vi "Advanced VI Analysis.vi"() -> ()   [LabVIEW 2023]
doc: "This example uses the advanced VI Analyzer VIs to perform an analysis on an LLB of VIs. The \"New Task\" VI uses preset test settings loaded from a CFG file that was created from the VI Analyzer user interface. Certain advanced VIs are used to perform tasks like adding an LLB to the analysis, removing a single VI from the analysis, removing certain tests from the analysis, and modifying a configuration value on one test. Once the analysis performed by \"VIAn Run.vi\" is complete, the \"VIAn Easy Report.vi\" saves the analysis results to an HTML report."
uses:
  <vilib>/Platform/browser.llb/Open URL in Default Browser (path).vi
  <vilib>/addons/analyzer/NI_VIAnalyzerTKVIs.lvlib
panel:
  in  "Tests with ten maximum failures":string[](array[string])=["Coercion Dots", "Spell Check"]
  out "VI in Analysis":string
  out "Analysis Progress":dbl(slide) scale=0.0..100.0
  out "Tests Run":string[](array[string])
  out "VIs Tested":path[](array[path])
  in  "Modified Value":T1={"Test Name"="VI Documentation", "Control Name"="Control Description", "Control Value"=FALSE}
  in  "VI to Remove":string="Container VI.vi"
  in  "Excluded Tests":string[](array[string])=["Enabled Debugging", "Panel Size and Position"]
  # "Overview: Demonstrates the use of the VI Analyzer and VI Analyzer Utility VIs to customize a programmatic analysis.\nRequirements: VI Analyzer Toolkit\nInstructions:\nRun the VI."
  # "Exclude these tests from the VI Analyzer Task."
  # "Set these tests to have 10 maximum failures for the VI Analyzer Task."
  # "Remove the top-level placeholder VI from the analysis."
  # "Disable the option on the \"VI Documentation\" test to analyze control descriptions."
  # "Show the progress of the analysis."
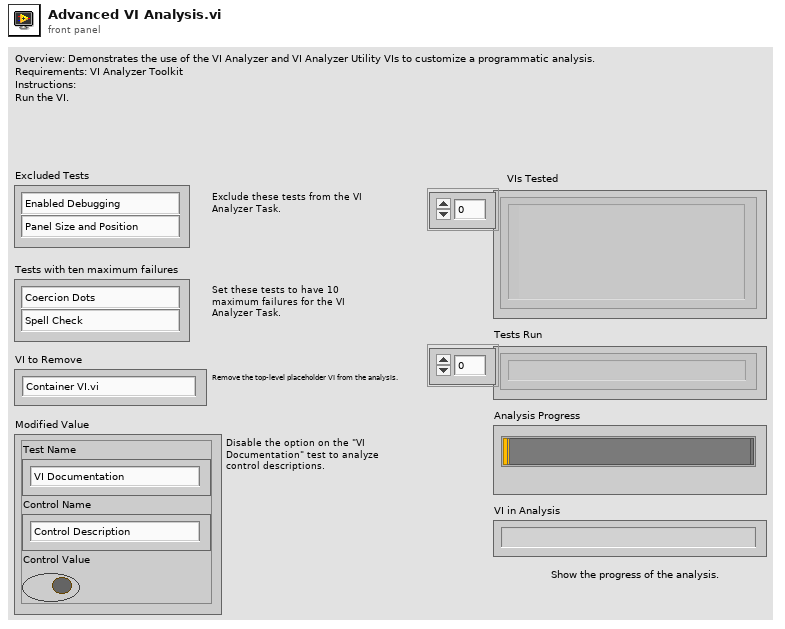
[diagram p1: front panel]
types:
  T1 = cluster{"Test Name":string, "Control Name":string, "Control Value":bool}
  T2 = typedef "VIAnAPI Ref.ctl" = refnum<k1>
  T3 = typedef "VIAnCtl API Test Config Data.ctl" = cluster{"Test Ranking":T4, "Max Failures":u32, "Control Values":T5[], "Run Test?":bool}
  T4 = typedef "VIAnCtl TestRanking.ctl" = u16
  T5 = typedef "VIAnCtl Config Control Value.ctl" = cluster{"Control Name":string, "Control Value":variant}
  T6 = typedef "VIAnCtl Results.ctl" = cluster{"Test Name":string, "Results Data":T7[], "Status":T8, "Exceed Max Fails?":bool}
  T7 = typedef "VIAnCtl ResultsData (index).ctl" = cluster{"Result Message":string, "Ref Index":i32}
  T8 = typedef "VIAnCtl ResultStatus.ctl" = enum16{"Pass", "Fail", "Skipped", "VI not loadable", "Test not loadable", "Test not runnable", "Test error out"}
  T9 = typedef "VIAnRes Parsed Results Data (by VI).ctl" = cluster{"VI Path":path, "Pass":cluster{"row":i32, "column":i32}[], "Fail":cluster{"row":i32, "column":i32}[], "Skipped":cluster{"row":i32, "column":i32}[], "VI not loadable":cluster{"row":i32, "column":i32}[], "Test not loadable":cluster{"row":i32, "column":i32}[], "Test not runnable":cluster{"row":i32, "column":i32}[], "Test error out":cluster{"row":i32, "column":i32}[]}
  T10 = typedef "VIAnRes Parsed Results Data (by Test).ctl" = cluster{"Test Name":string, "Pass":cluster{"VI Path":path, "index":cluster{"row":i32, "column":i32}}[], "Fail":cluster{"VI Path":path, "index":cluster{"row":i32, "column":i32}}[], "Skipped":cluster{"VI Path":path, "index":cluster{"row":i32, "column":i32}}[]}
  T11 = typedef "VIAnCtl Test Config Data.ctl" = cluster{"Test Name":string, "Config Ref":refnum<vi>, "Ref Valid?":bool, "Test Ranking":T4, "Max Failures":u32, "Test Path":path, "Control Values":T5[], "Selected?":bool}
  T12 = cluster{"Raw Results":T6[][], "Parsed Results Data (by VI)":T9[], "Parsed Results Data (by Test)":T10[], "Summary Statistics":cluster{"Passed Tests":i32, "Failed Tests":i32, "Skipped Tests":i32, "VIs not loadable":i32, "Tests not loadable":i32, "Tests not runnable":i32, "Test error out":i32, "Start Time":u32, "Total Time (s)":dbl}, "Test Config Data":T11[]}
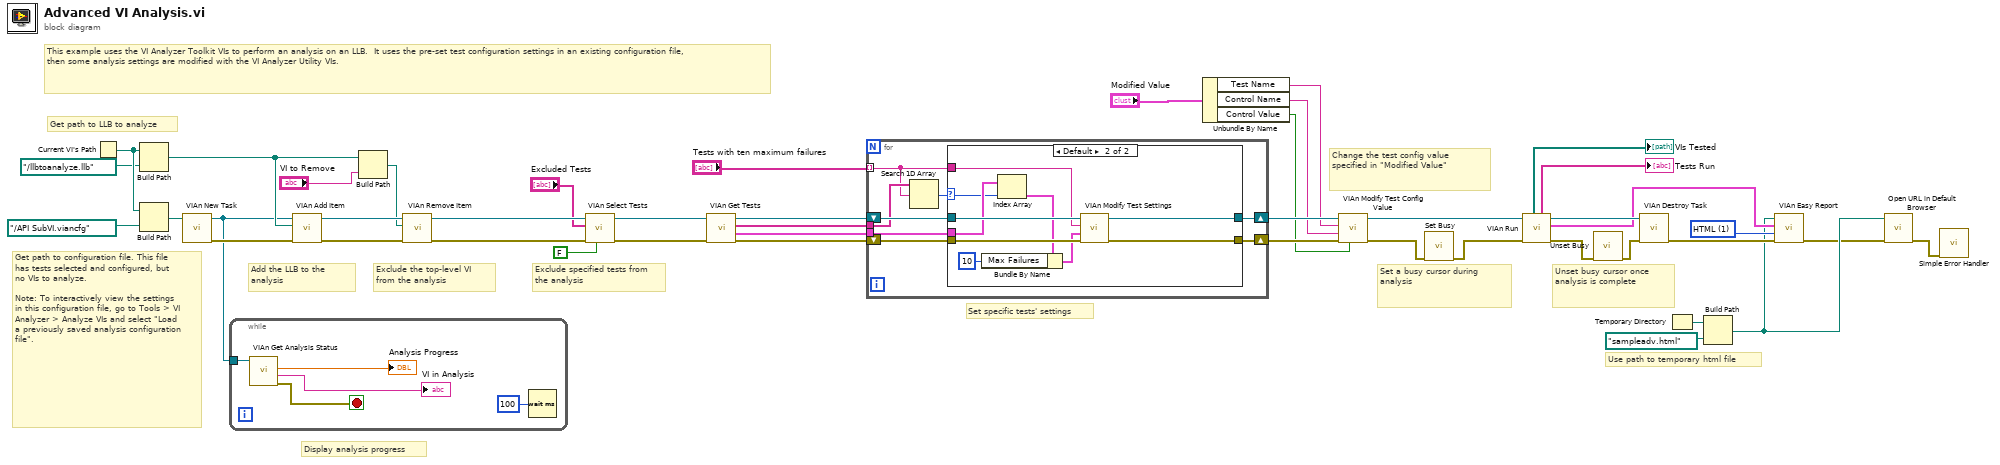
[diagram p0: block diagram]
diagram:
  w32 = u16 1 items=["ASCII", "HTML", "RSL File"] ("Report Save Type (ASCII)")
  # "Set specific tests' settings"
  # "Exclude specified tests from the analysis"
  # "Display analysis progress"
  # "Unset busy cursor once analysis is complete"
  # "Set a busy cursor during analysis"
  # "Get path to LLB to analyze"
  # "This example uses the VI Analyzer Toolkit VIs to perform an analysis on an LLB.  It uses the pre-set test configuration settings in an existing configuration file, then some analysis settings are modified with the VI Analyzer Utility VIs."
  # "Use path to temporary html file"
  # "Change the test config value specified in \"Modified Value\""
  # "Get path to configuration file. This file has tests selected and configured, but no VIs to analyze.\n\nNote: To interactively view the settings in this configuration file, go to Tools > VI Analyzer > Analyze VIs and select \"Load a previously saved analysis configuration file\"."
  # "Exclude the top-level VI from the analysis"
  # "Add the LLB to the analysis"
  n1 = Current VI's Path() -> (path=w41:path)
  n2 = Build Path(base path=w41, name or relative path=path "../llbtoanalyze.llb" ("path")) -> (appended path=w37:path)
  n3 = Build Path(base path=w41, name or relative path=path "../API SubVI.viancfg" ("path")) -> (appended path=w44:path)
  n4 = call <vilib>:"VIAn New Task.vi"("Path to Configuration File"=w44) -> ("error out"=w42:errorcluster, "VI Analyzer Task"=w15:T2)  [unwired: 2 in, 7 out]
  n5 = while {
    tunnel: w15 -> [w49]
    stop <- w45 stop-if-true
    n6 = call <vilib>:"VIAn Get Analysis Status.vi"("VI Analyzer Task in"=w49) -> ("error out"=w45:errorcluster, "VI in Analysis"=→"VI in Analysis":string, "Percent Complete"=→"Analysis Progress":dbl)  [unwired: 1 in, 7 out]
    n7 = Wait (ms)(milliseconds to wait=u32 100) -> ()  [unwired: 1 out]
  }
  n8 = call <vilib>:"VIAn Add Item.vi"("error in (no error)"=w42, "Item to Add"=w37, "VI Analyzer Task in"=w15) -> ("error out"=w38:errorcluster, "VI Analyzer Task out"=w39:T2)  [unwired: 7 out]
  n9 = Build Path(base path=w37, name or relative path="VI to Remove") -> (appended path=w36:path)
  n10 = call <vilib>:"VIAn Remove Item.vi"("error in (no error)"=w38, "Item to Remove"=w36, "VI Analyzer Task in"=w39) -> ("error out"=w12:errorcluster, "VI Analyzer Task out"=w14:T2)  [unwired: 7 out]
  n11 = call <vilib>:"VIAn Select Tests.vi"("Select Test? (T)"=FALSE, "error in (no error)"=w12, "Test Names"="Excluded Tests", "VI Analyzer Task in"=w14) -> ("error out"=w9:errorcluster, "VI Analyzer Task out"=w10:T2)  [unwired: 6 out]
  n12 = call <vilib>:"VIAn Get Tests.vi"("error in (no error)"=w9, "VI Analyzer Task in"=w10) -> ("error out"=w8:errorcluster, "Test Configurations"=w6:T3[], "Test Names"=w5:string[], "VI Analyzer Task out"=w7:T2)  [unwired: 6 out]
  n13 = for {
    shift-right: [w54] -> w30
    shift-left: w8 -> [w56]
    shift-right: [w55] -> w31
    shift-left: w7 -> [w57]
    tunnel: "Tests with ten maximum failures" -> [w52] mode=indexing
    tunnel: w6 -> [w50]
    tunnel: w5 -> [w53]
    n14 = Search 1D Array(1D array=w53, element=w52) -> (index of element=w51:i32)  [unwired: 1 out]
    n15 = case shown="Default" w51 {
      selector: w51 -> [_ w62]
      tunnel: w57 -> [w59 w69]
      tunnel: w56 -> [w58 w68]
      tunnel: [w59 w67] -> w55
      tunnel: [w58 w66] -> w54
      tunnel: w52 -> [_ w64]
      tunnel: w50 -> [_ w63]
      frame -1 {
      }
      frame Default {
        n16 = Index Array(array=w63, index=w62) -> (element=w61:T3)
        n17 = Bundle By Name(cluster=w61, "Max Failures"=u32 10) -> (w65:T3)
        n18 = call <vilib>:"VIAn Modify Test Settings.vi"("error in (no error)"=w68, "New Test Info"=w65, "Test Name"=w64, "VI Analyzer Task in"=w69) -> ("error out"=w66:errorcluster, "VI Analyzer Task out"=w67:T2)  [unwired: 6 out]
      }
    }
  }
  n19 = Unbundle By Name("Modified Value") -> ("Test Name"=w27:string, "Control Name"=w26:string, "Control Value"=w25:bool)
  n20 = call <vilib>:"VIAn Modify Test Config Value.vi"("Control Value"=w25, "error in (no error)"=w30, "Control Name"=w26, "Test Name"=w27, "VI Analyzer Task in"=w31) -> ("error out"=w19:errorcluster, "VI Analyzer Task out"=w20:T2)  [unwired: 5 out]
  n21 = call <vilib>:"Set Busy.vi"("error in (no error)"=w19) -> ("error out"=w18:errorcluster)  [unwired: 3 in, 7 out]
  n22 = call <vilib>:"VIAn Run.vi"("error in (no error)"=w18, "VI Analyzer Task in"=w20) -> ("error out"=w17:errorcluster, "Analysis Results"=w33:T12, "VI Analyzer Task out"=w35:T2, "Tests Run"=→"Tests Run":string[], "VIs Tested"=→"VIs Tested":path[])  [unwired: 5 out]
  n23 = call <vilib>:"Unset Busy.vi"("error in (no error)"=w17) -> ("error out"=w16:errorcluster)  [unwired: 1 in, 9 out]
  n24 = call <vilib>:"VIAn Destroy Task.vi"("error in (no error)"=w16, "VI Analyzer Task in"=w35) -> ("error out"=w34:errorcluster)  [unwired: 9 out]
  n25 = Temporary Directory() -> (w24:path)
  n26 = Build Path(base path=w24, name or relative path=path "sampleadv.html" ("path")) -> (appended path=w3:path)
  n27 = call <vilib>:"VIAn Easy Report.vi"("error in (no error)"=w34, "Report Save Type (ASCII)"=w32, "Analysis Results"=w33, "Report Save Path"=w3) -> ("error out"=w2:errorcluster)  [unwired: 3 in, 4 out]
  n28 = call-poly <vilib>:"Open URL in Default Browser.vi"("error in (no error)"=w2, "path"=w3) -> ("error out"=w1:errorcluster)  [unwired: 5 out]
  n29 = call <vilib>:"Simple Error Handler.vi"("error in (no error)"=w1) -> ()  [unwired: 4 in, 5 out]
